vi "VisionAlign.vi"(8 "Error In":errorcluster) -> (0 "Error Out":errorcluster)   [LabVIEW 2016]
uses:
  <vilib>/Rock Robotics/Network Tables/NT Read Number.vi
  <vilib>/addons/control/pid/pid.llb/PID (DBL).vi
  <vilib>/addons/control/pid/NI_PID_pid.lvlib
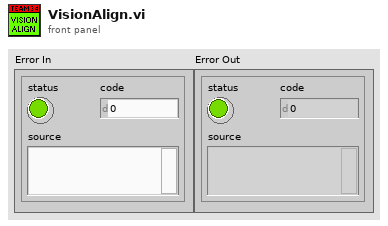
[diagram p1: front panel]
types:
  T1 = typedef "WPI_GyroDevRef.ctl" = cluster{"DevStatus":errorcluster, "Analog Channel":T2, "Offset":dbl, "Gain (VoltsPerDegree/Second)":dbl, "Gyro Type":enum16{"Analog", "XRS450"}, "Handle":i32, "SPI Bus":T3, "Device Found":bool, "Sample Rate":dbl, "Calibrate On Open":bool}
  T2 = typedef "FPGA_AIChannel.ctl" = enum8{"AI 0", "AI 1", "AI 2", "AI 3", "AI MXP 0", "AI MXP 1", "AI MXP 2", "AI MXP 3", "Invalid"}
  T3 = typedef "spi_bus.ctl" = enum16{"SPI On-Board, CS0", "SPI On-Board, CS1", "SPI On-Board, CS2", "SPI On-Board, CS3", "SPI MXP", "Invalid"}
  T4 = cluster{"proportional gain (Kc)":dbl, "integral time (Ti, min)":dbl, "derivative time (Td, min)":dbl}
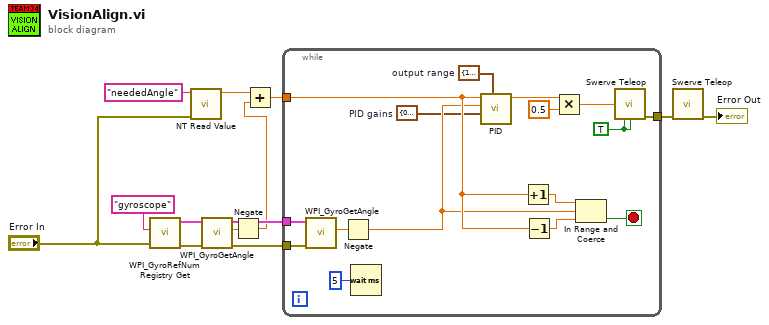
[diagram p0: block diagram]
diagram:
  n1 = call <vilib>:"WPI_GyroRefNum Registry Get.vi"("error in (no error)"="Error In", "refnum name"="gyroscope") -> ("error out"=w6:errorcluster, "GyroDevRef"=w7:T1)  [unwired: 8 in]
  n2 = call-poly <vilib>:"NT Read Value.vi"("error in"="Error In", "Name"="neededAngle") -> ("Numeric"=w9:dbl)  [unwired: 8 in, 1 out]
  n3 = call <vilib>:"WPI_GyroGetAngle.vi"("error in"=w6, "GyroDevRef"=w7) -> ("error out"=w13:errorcluster, "Angle"=w10:dbl, "GyroDevRef"=w12:T1)  [unwired: 5 in, 2 out]
  n4 = Negate(x=w10) -> (-x=w11:dbl)
  n5 = Add(x=w9, y=w11) -> (x+y=w4:dbl)
  n6 = while {
    tunnel: w4 -> [w20]
    tunnel: [w25] -> w5
    tunnel: w12 -> [w19]
    tunnel: w13 -> [w18]
    stop <- w29 stop-if-true
    w14 = cluster{"output high":dbl, "output low":dbl} {"output high"=1.0, "output low"=-1.0}  # output range
    w15 = T4 {"proportional gain (Kc)"=0.04, "integral time (Ti, min)"=0.0, "derivative time (Td, min)"=0.0}  # PID gains
    w24 = TRUE ("Robot Centric?")
    n7 = call <vilib>:"WPI_GyroGetAngle.vi"("error in"=w18, "GyroDevRef"=w19) -> ("Angle"=w17:dbl)  [unwired: 5 in, 4 out]
    n8 = Negate(x=w17) -> (-x=w16:dbl)
    n9 = Wait (ms)(milliseconds to wait=u32 5) -> ()  [unwired: 1 out]
    n10 = call-poly <vilib>:"PID.vi"("output range"=w14, "PID gains"=w15, "process variable"=w16, "setpoint"=w20) -> ("output"=w28:dbl)  [unwired: 6 in, 1 out]
    n11 = Increment(x=w20) -> (x+1=w23:dbl)
    n12 = Decrement(x=w20) -> (x-1=w22:dbl)
    n13 = Multiply(x=w28, y=0.5) -> (x*y=w26:dbl)
    n14 = In Range and Coerce(upper limit=w23, x=w16, lower limit=w22) -> (In Range?=w29:bool)  [unwired: 1 out]
    n15 = call "Swerve Teleop.vi"("Z"=w26, "Robot Centric?"=w24, "Autonomous?"=w24) -> ("Error Out"=w25:errorcluster)  [unwired: 8 in, 4 out]
  }
  n16 = call "Swerve Teleop.vi"("Error In"=w5) -> ("Error Out"=→"Error Out":errorcluster)  [unwired: 10 in, 4 out]
